vi "Impedance Control.vi"(0 "PID On":bool) -> (5 "Total (V)":dbl[](array[slide]) scale=-8.0..8.0, 6 "Force (N)":T3(graph)={"M1 ref force"=20.0, "M2 ref force"=10.768311870905725, "M1 mes force"=3.690819426740976, "M2 mes force"=4.004504201458466})   [LabVIEW 2021]
uses:
  <vilib>/Platform/TimedLoop/XDataNode/timing_clust.ctl
  <vilib>/Platform/TimedLoop/XDataNode/nitl_modes.ctl
  <vilib>/Platform/TimedLoop/XDataNode/wakeup.ctl
  <vilib>/DAQmx/write.llb/DAQmx Write (Digital 1D Bool 1Chan 1Samp).vi
  <vilib>/DAQmx/write.llb/DAQmx Write (Analog 1D DBL NChan 1Samp).vi
  <vilib>/DAQmx/create/channels.llb/DAQmx Create Channel (DO-Digital Output).vi
  <vilib>/DAQmx/create/channels.llb/DAQmx Create Channel (AO-Voltage-Basic).vi
  <vilib>/DAQmx/create/channels.llb/DAQmx Create Channel (AI-Voltage-Basic).vi
  <vilib>/addons/control/pid/pid.llb/PID (DBL).vi
  <vilib>/DAQmx/miscellaneous.llb/DAQmx Fill In Error Info.vi
  <vilib>/Platform/TimedLoop/XDataNode/XDataNode.xnode
  <vilib>/Platform/TimedLoop/XDataNode/XDNodeRunTimeDep.lvlib
  <vilib>/addons/control/pid/NI_PID_pid.lvlib
panel:
  out "In Range? 2":bool
  in  "PID gains":T1={"proportional gain (Kc)"=0.15, "integral time (Ti, min)"=0.0, "derivative time (Td, min)"=0.0} {"derivative time (Td, min)" format="%.3f"; "integral time (Ti, min)" format="%.3f"; "proportional gain (Kc)" format="%.3f"}
  out "output":dbl(slide)=-9.231688129094275 scale=-40.0..40.0
  out "Boolean":bool=TRUE
  in  "Numeric":dbl=3.0
  in  "Tab Control":enum32{"PID Gain", "PIN On"}(tab)=enum."PIN On"
  in  "Gains":T2(array[cluster])=[{"proportional gain (Kc)"=0.17, "integral time (Ti, min)"=0.0, "derivative time (Td, min)"=0.0}, {"proportional gain (Kc)"=0.17, "integral time (Ti, min)"=0.0, "derivative time (Td, min)"=0.0}] {"derivative time (Td, min)" format="%.3f"; "integral time (Ti, min)" format="%.3f"; "proportional gain (Kc)" format="%.3f"}
  out "PID (V)":dbl[](array[slide])=[2.7725606974540344, 1.0] scale=-8.0..8.0
  out "Trigger":bool
  out "Position (mm)":cluster{"Position":dbl, "ref_x (mm)":dbl}(graph)={"Position"=61.544587527295164, "ref_x (mm)"=0.0}
  in  "Loadcell":bool
  in  "Encoder":bool
  out "In Range?":bool
  out "Speed (RPM)":dbl[](array[knob]) scale=-200.0..200.0
  out "time (s)":dbl=637.168
  in  "Set Point":dbl(slide)=19.690402476780186 scale=0.0..40.0
  in  "Motor Enable":bool[](array[boolean])=[FALSE, FALSE]
  in  "stop":bool
  # "FORCE"
  # "TRAJECTORY"
  # "INITIALIZE"
  # "TUNE"
  # "MONITOR"
  # "DEVEL"
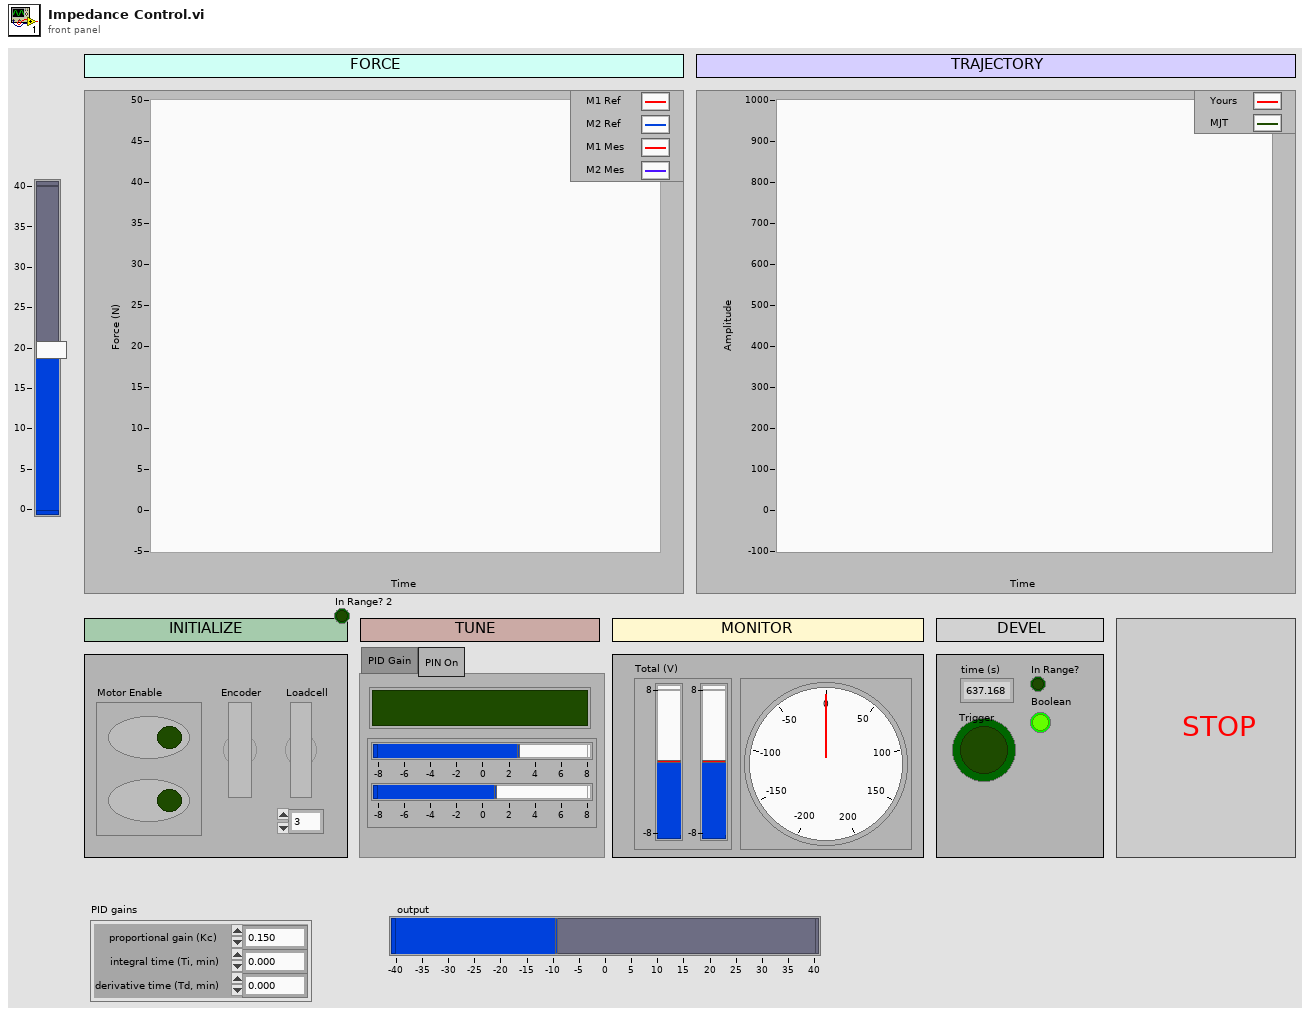
[diagram p1: front panel]
types:
  T1 = cluster{"proportional gain (Kc)":dbl, "integral time (Ti, min)":dbl, "derivative time (Td, min)":dbl}
  T2 = cluster{"proportional gain (Kc)":dbl, "integral time (Ti, min)":dbl, "derivative time (Td, min)":dbl}[]
  T3 = cluster{"M1 ref force":dbl, "M2 ref force":dbl, "M1 mes force":dbl, "M2 mes force":dbl}
  T4 = typedef "XDNodeRunTimeDep.lvlib/timing_clust.ctl" = cluster{"Expected End [f-1]":u64, "Actual End [f-1]":u64, "Finished Late? [f-1]":bool, "Expected End [i-1]":u64, "Actual End [i-1]":u64, "Finished Late? [i-1]":bool, "Expected Start [i]":u64, "Actual Start [i]":u64, "Expected Start [f]":u64, "Actual Start [f]":u64, "Source Name":string, "Structure Name":string, "Period":i64, "Deadline":i64, "Offset":i64, "Start":i64, "Priority":i32, "Timeout":i32, "Mode":T5, "Wakeup Reason":T6, "Error":errorcluster, "Source Type":string, "Secondary Source Type":string, "Global End Time":u64, "Global Start Time":u64, "Frame Duration":u64, "Iteration Duration":u64, "Assigned CPU":i32, "I/O Scan Engine Mode":u32}
  T5 = typedef "XDNodeRunTimeDep.lvlib/nitl_modes.ctl" = enum32{"No Change", "Process missed periods, maintain original phase", "Discard missed periods, maintain original phase", "Process missed periods, ignore original phase", "Discard missed periods, ignore original phase"}
  T6 = typedef "XDNodeRunTimeDep.lvlib/wakeup.ctl" = enum32{"Normal", "Aborted", "Asynchronous wakeup", "Timing source error", "Timed loop error", "Timeout"}
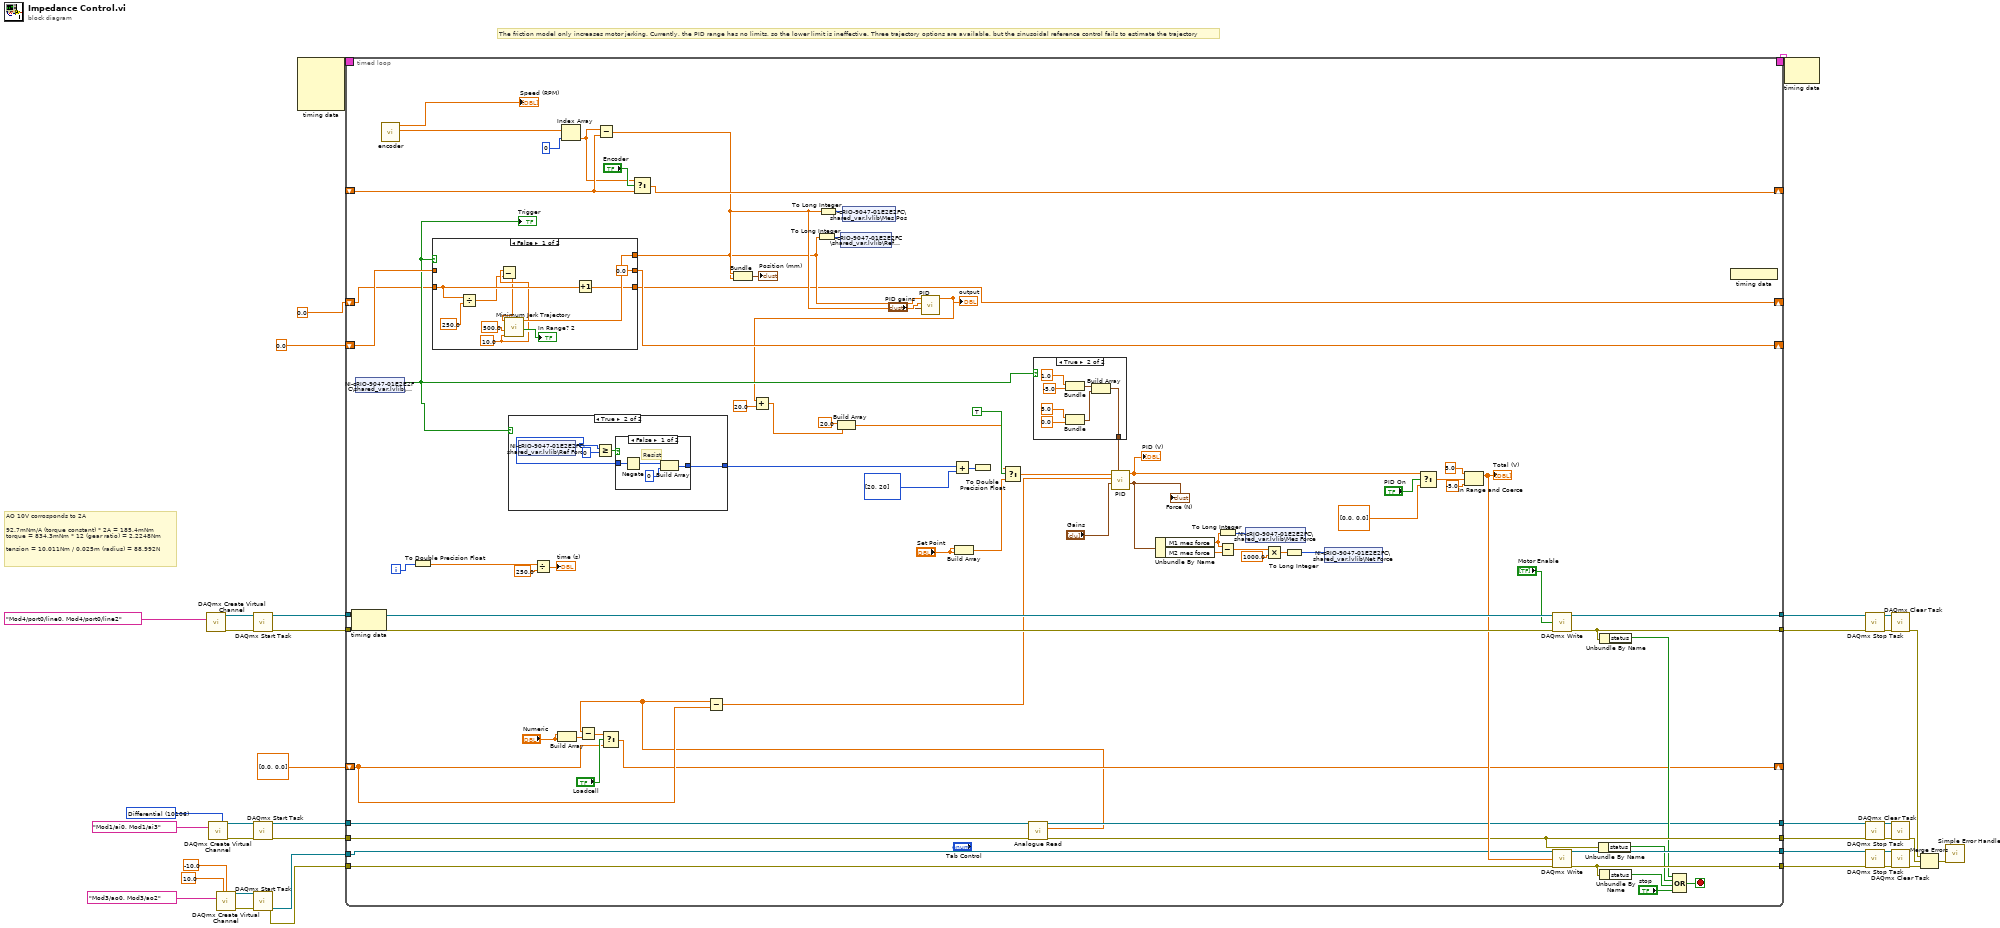
[diagram p0: block diagram]
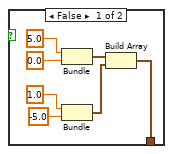
[diagram p2: hidden frame]
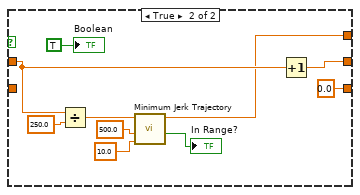
[diagram p3: hidden frame]
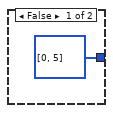
[diagram p4: hidden frame]
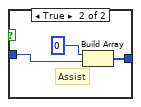
[diagram p5: hidden frame]
diagram:
  w4 = 10106 items=["Default"=-1, "RSE"=10083, "NRSE"=10078, "Differential"=10106, "Pseudodifferential"=12529] ("input terminal configuration")
  # "The friction model only increases motor jerking. Currently, the PID range has no limits, so the lower limit is ineffective. Three trajectory options are available, but the sinusoidal reference control fails to estimate the trajectory"
  # "AO 10V corrosponds to 2A\n\n92.7mNm/A (torque constant) * 2A = 185.4mNm\ntorque = 834.3mNm * 12 (gear ratio) = 2.2248Nm\n\ntension = 10.011Nm / 0.025m (radius) = 88.992N"
  n1 = call-poly <vilib>:"DAQmx Create Virtual Channel.vi"("lines"=tag "Mod4/port0/line0, Mod4/port0/line2") -> ("task out"=w31:refnum<k21>, "error out"=w30:errorcluster)  [unwired: 13 in]
  n2 = call-poly <vilib>:"DAQmx Create Virtual Channel.vi"("input terminal configuration"=w4, "physical channels"=tag "Mod1/ai0, Mod1/ai3") -> ("task out"=w21:refnum<k21>, "error out"=w22:errorcluster)  [unwired: 12 in]
  n3 = call-poly <vilib>:"DAQmx Create Virtual Channel.vi"("maximum value"=10.0 ("AO max"), "minimum value"=-10.0 ("AO min"), "physical channels"=tag "Mod3/ao0, Mod3/ao2" ("Physical Channel(s)")) -> ("task out"=w15:refnum<k21>, "error out"=w14:errorcluster)  [unwired: 11 in]
  n4 = call <vilib>:"DAQmx Start Task.vi"("task/channels in"=w31, "error in"=w30) -> ("task out"=w28:refnum<k21>, "error out"=w27:errorcluster)  [unwired: 12 in]
  n5 = call <vilib>:"DAQmx Start Task.vi"("task/channels in"=w21, "error in"=w22) -> ("task out"=w19:refnum<k21>, "error out"=w18:errorcluster)  [unwired: 12 in]
  n6 = call <vilib>:"DAQmx Start Task.vi"("task/channels in"=w15, "error in"=w14) -> ("task out"=w33:refnum<k21>, "error out"=w32:errorcluster)  [unwired: 12 in]
  n7 = node-c288() -> (w35:T4)  [unwired: 4 in]
  n8 = timed-loop {
    tunnel: [w116] -> w39
    tunnel: [w115] -> w38
    tunnel: [w73] -> w37
    tunnel: [w102] -> w36
    tunnel: w19 -> [w113]
    timing: w35 -> [_]
    timing-out: [_] -> w34
    tunnel: w18 -> [w112]
    tunnel: w33 -> [w72]
    tunnel: w32 -> [w114]
    tunnel: w28 -> [w111]
    tunnel: w27 -> [w110]
    tunnel: [w109] -> w24
    tunnel: [w103] -> w23
    shift-right: [w84] -> _
    shift-left: 0.0 ("total time") -> [w85]
    shift-right: [w79] -> _
    shift-left: _ -> [w77]
    shift-right: [w61] -> _
    shift-left: dbl[] [0.0, 0.0] ("measured force") -> [w62]
    shift-right: [w45] -> _
    shift-left: 0.0 ("total time") -> [w46]
    i -> [w90]
    stop <- w98 stop-if-true
    n9 = node-c288() -> ()  [unwired: 1 in, 1 out]
    n10 = shared-variable "NI-cRIO-9047-01E2E2FC\\shared_var.lvlib\\Trigger"() -> (w54:bool)  [unwired: 1 in, 1 out]
    "Trigger" <- w54
    n11 = call "encoder.vi"() -> ("Mes Pos (mm)"=w82:dbl[], "RPM"=→"Speed (RPM)":dbl[])  [unwired: 10 in]
    n12 = To Double Precision Float(number=w90) -> (double precision float=w89:dbl)
    n13 = case shown="False" w54 {
      tunnel: w85 -> [_ w146]
      tunnel: [0.0 w149] -> w84
      tunnel: [w139 w145] -> w48
      tunnel: w46 -> [w136 _]
      tunnel: [w137 0.0] -> w45
      frame False {
        w135 = 10.0 ("total time")
        n14 = Divide(x=w136, y=250.0) -> (x/y=w134:dbl)
        n15 = Subtract(x=w135, y=w134) -> (x-y=w133:dbl)
        n16 = call "Minimum Jerk Trajectory.vi"("total time"=w135, "total length"=500.0, "t (sec)"=w133) -> ("In Range?"=→"In Range? 2":bool, "ref_x (mm)"=w139:dbl)  [unwired: 7 in]
        n17 = Increment(x=w136) -> (x+1=w137:dbl)
      }
      frame True {
        n18 = Divide(x=w146, y=250.0) -> (x/y=w147:dbl)
        n19 = call "Minimum Jerk Trajectory.vi"("total time"=10.0, "total length"=500.0, "t (sec)"=w147) -> ("In Range?"=→"In Range?":bool, "ref_x (mm)"=w145:dbl)  [unwired: 7 in]
        n20 = Increment(x=w146) -> (x+1=w149:dbl)
        "Boolean" <- TRUE ("Boolean")
      }
    }
    n21 = case shown="True" w54 {
      tunnel: [i32[] [0, 5] w157] -> w75
      frame False {
      }
      frame True {
        n22 = shared-variable "NI-cRIO-9047-01E2E2FC\\shared_var.lvlib\\Ref Force"() -> (w156:i32)  [unwired: 1 in, 1 out]
        n23 = Greater Or Equal?(x=w156, y=0) -> (x >= y?=w154:bool)
        n24 = case shown="False" w154 {
          tunnel: w156 -> [w160 w163]
          tunnel: [w161 w164] -> w157
          frame False {
            # "Resist"
            n25 = Negate(x=w160) -> (-x=w158:i32)
            n26 = Build Array(w158, 0 ("element")) -> (w161:i32[])
          }
          frame True {
            # "Assist"
            n27 = Build Array(0 ("element"), w163) -> (w164:i32[])
          }
        }
      }
    }
    n28 = Divide(x=w89, y=250.0) -> (x/y=→"time (s)":dbl)
    n29 = Build Array("Numeric", "Numeric") -> (w50:dbl[])
    n30 = Index Array(array=w82, index=0) -> (element=w76:dbl)
    n31 = Subtract(x=w76, y=w77) -> (x-y=w49:dbl)
    n32 = Select(t=w76, s="Encoder", f=w77) -> (s? t:f=w79:dbl)
    n33 = Bundle(w49, "ref_x (mm)"=w48) -> (→"Position (mm)":cluster{dbl, "ref_x (mm)":dbl})  [unwired: 1 in]
    n34 = To Long Integer(number=w48) -> (32bit integer=w57:i32)
    n35 = To Long Integer(number=w49) -> (32bit integer=w56:i32)
    n36 = shared-variable "NI-cRIO-9047-01E2E2FC\\shared_var.lvlib\\Ref Pos"(w57) -> ()  [unwired: 1 in, 1 out]
    n37 = shared-variable "NI-cRIO-9047-01E2E2FC\\shared_var.lvlib\\Mes Pos"(w56) -> ()  [unwired: 1 in, 1 out]
    n38 = call-poly <vilib>:"PID.vi"("PID gains"="PID gains", "process variable"=w49, "setpoint"=w48) -> ("output"=w42:dbl)  [unwired: 7 in, 1 out]
    "output" <- w42
    n39 = Add(x=w42, y=20.0) -> (x+y=w41:dbl)
    n40 = Build Array(20.0 ("element"), w41) -> (w40:dbl[])
    n41 = Add(x=w75, y=i32[] [20, 20] ("x")) -> (x+y=w71:i32[])
    n42 = Build Array("Set Point", "Set Point") -> (w92:dbl[])
    n43 = To Double Precision Float(number=w71) -> ()  [unwired: 1 out]
    n44 = Select(t=w40, s=TRUE, f=w92) -> (s? t:f=w68:dbl[])
    n45 = call "Analogue Read.vi"("error in"=w112, "task/channels in"=w113) -> ("error out"=w102:errorcluster, "measured force"=w59:dbl[], "task out"=w73:refnum<k21>)  [unwired: 6 in, 1 out]
    n46 = Subtract(x=w59, y=w50) -> (x-y=w58:dbl[])
    n47 = Select(t=w58, s="Loadcell", f=w62) -> (s? t:f=w61:dbl[])
    n48 = Subtract(x=w59, y=w62) -> (x-y=w60:dbl[])
    n49 = case shown="True" w54 {
      tunnel: [w119 w126] -> w64
      frame False {
        n50 = Bundle(5.0, 0.0) -> (w125:cluster{dbl, dbl})  [unwired: 1 in]
        n51 = Bundle(1.0, -5.0) -> (w124:cluster{dbl, dbl})  [unwired: 1 in]
        n52 = Build Array(w125, w124) -> (w119:cluster{dbl, dbl}[])
      }
      frame True {
        n53 = Bundle(1.0, -5.0) -> (w127:cluster{dbl, dbl})  [unwired: 1 in]
        n54 = Bundle(5.0, 0.0) -> (w128:cluster{dbl, dbl})  [unwired: 1 in]
        n55 = Build Array(w127, w128) -> (w126:cluster{dbl, dbl}[])
      }
    }
    n56 = call <vilib>:"PID.vi"("output range"=w64, "PID gains"="Gains", "mes force"=w60, "ref force"=w68) -> ("output cluster"=w52:T3, "PID output"=w96:dbl[])  [unwired: 6 in]
    "Force (N)" <- w52
    "PID (V)" <- w96
    n57 = Unbundle By Name(w52) -> ("M1 mes force"=w65:dbl, "M2 mes force"=w66:dbl)
    n58 = To Long Integer(number=w65) -> (32bit integer=w67:i32)
    n59 = Subtract(x=w65, y=w66) -> (x-y=w70:dbl)
    n60 = shared-variable "NI-cRIO-9047-01E2E2FC\\shared_var.lvlib\\Mes Force"(w67) -> ()  [unwired: 1 in, 1 out]
    n61 = Multiply(x=w70, y=1000.0) -> (x*y=w53:dbl)
    n62 = To Long Integer(number=w53) -> (32bit integer=w55:i32)
    n63 = shared-variable "NI-cRIO-9047-01E2E2FC\\shared_var.lvlib\\Net Force"(w55) -> ()  [unwired: 1 in, 1 out]
    n64 = Select(t=w96, s="PID On", f=dbl[] [0.0, 0.0]) -> (s? t:f=w94:dbl[])
    n65 = In Range and Coerce(upper limit=5.0, x=w94, lower limit=-5.0) -> (coerced(x)=w104:dbl[])  [unwired: 1 out]
    "Total (V)" <- w104
    n66 = call-poly <vilib>:"DAQmx Write.vi"("task/channels in"=w111, "data"="Motor Enable", "error in"=w110) -> ("task out"=w109:refnum<k21>, "error out"=w103:errorcluster)  [unwired: 10 in, 1 out]
    n67 = call-poly <vilib>:"DAQmx Write.vi"("task/channels in"=w72, "data"=w104, "error in"=w114) -> ("task out"=w116:refnum<k21>, "error out"=w115:errorcluster)  [unwired: 10 in, 1 out]
    n68 = Unbundle By Name(w102) -> ("status"=w100:bool)
    n69 = Unbundle By Name(w103) -> ("status"=w99:bool)
    n70 = Unbundle By Name(w115) -> ("status"=w101:bool)
    n71 = Compound Arithmetic op=OR(w99, w100, w101, "stop") -> (w98:bool)
    n72 = node-c288() -> ()  [unwired: 1 out]
  }
  n73 = node-c288(w34) -> ()  [unwired: 1 out]
  n74 = call <vilib>:"DAQmx Stop Task.vi"("task/channels in"=w24, "error in"=w23) -> ("task out"=w26:refnum<k21>, "error out"=w25:errorcluster)  [unwired: 12 in]
  n75 = call <vilib>:"DAQmx Stop Task.vi"("task/channels in"=w37, "error in"=w36) -> ("task out"=w10:refnum<k21>, "error out"=w9:errorcluster)  [unwired: 12 in]
  n76 = call <vilib>:"DAQmx Stop Task.vi"("task/channels in"=w39, "error in"=w38) -> ("task out"=w12:refnum<k21>, "error out"=w11:errorcluster)  [unwired: 12 in]
  n77 = call <vilib>:"DAQmx Clear Task.vi"("task in"=w26, "error in"=w25) -> ("error out"=w5:errorcluster)  [unwired: 13 in]
  n78 = call <vilib>:"DAQmx Clear Task.vi"("task in"=w10, "error in"=w9) -> ("error out"=w6:errorcluster)  [unwired: 13 in]
  n79 = call <vilib>:"DAQmx Clear Task.vi"("task in"=w12, "error in"=w11) -> ("error out"=w7:errorcluster)  [unwired: 13 in]
  n80 = Merge Errors(w5, w6, w7) -> (w8:errorcluster)
  n81 = call <vilib>:"Simple Error Handler.vi"("error in (no error)"=w8) -> ()  [unwired: 4 in, 5 out]
